vi "test Create Map from Messages to Value Indexes.vi"(8 "error in (no error)":errorcluster, 11 "TestCase in":refnum<class "Engine.lvclass">) -> (0 "error out":errorcluster, 3 "TestCase out":refnum<class "Engine.lvclass">)   [LabVIEW 2020, in "Engine.lvclass"]
uses:
  Engine.lvclass
  Shared/1553 Channel.ctl
  Shared/Terminal Name and Address.ctl
  Shared/Address.ctl
  Shared/Message Definition.ctl
  Shared/Message Type.ctl
  Shared/Terminal Endpoint.ctl
  Shared/Parameter Definition.ctl
  Shared/Map of Messages to Value Indexes.ctl
  Shared/Message Map Key.ctl
  <vilib>/addons/_JKI Toolkits/VI Tester/TestCase.llb/TestCase.lvclass
  Engine/Custom Device/Custom Device.lvlib
  C:/Program Files (x86)/National Instruments/LabVIEW 2020/vi.lib/addons/_JKI Toolkits/VI Tester/TestCase.llb/TestCase.lvclass
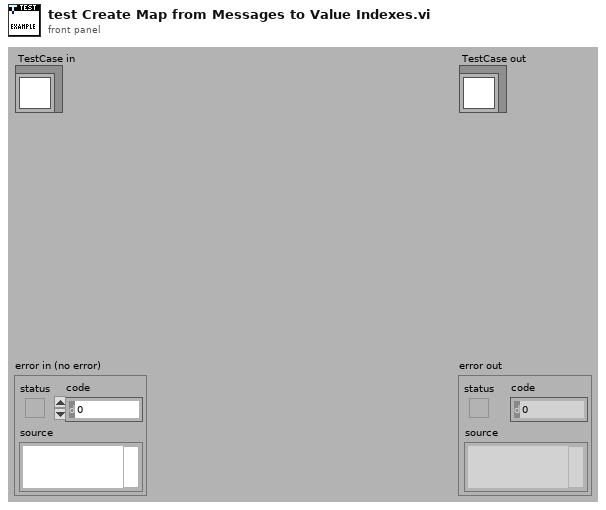
[diagram p1: front panel]
types:
  T1 = typedef "Map of Messages to Value Indexes.ctl" = map{T2, i32}
  T2 = typedef "Message Map Key.ctl" = cluster{"HW channel":u16, "terminal address":u16, "subaddress":u16, "mode code":u16}
  T3 = typedef "1553 Channel.ctl" = cluster{"HW channel":u16, "terminals":T4[], "messages":T6[], "acyclic frame names":string[]}
  T4 = typedef "Terminal Name and Address.ctl" = cluster{"name":string, "terminal address":T5}
  T5 = typedef "Address.ctl" = u16
  T6 = typedef "Message Definition.ctl" = cluster{"name":string, "message type":T7, "endpoint Rx":T8, "endpoint Tx":T8, "mode code":u16, "number of words":u16, "parameters":cluster{"name":string, "default value":dbl, "unit":string, "parameter definition":T9}[], "create timestamp channel":bool}
  T7 = typedef "Message Type.ctl" = string
  T8 = typedef "Terminal Endpoint.ctl" = cluster{"terminal address":T5, "subaddress":T5}
  T9 = typedef "Parameter Definition.ctl" = cluster{"start index":i32, "size (bits)":i32, "encoding":enum16{"BNR", "BCD", "Discrete"}, "signed":bool, "multiplier":dbl, "offset":dbl}
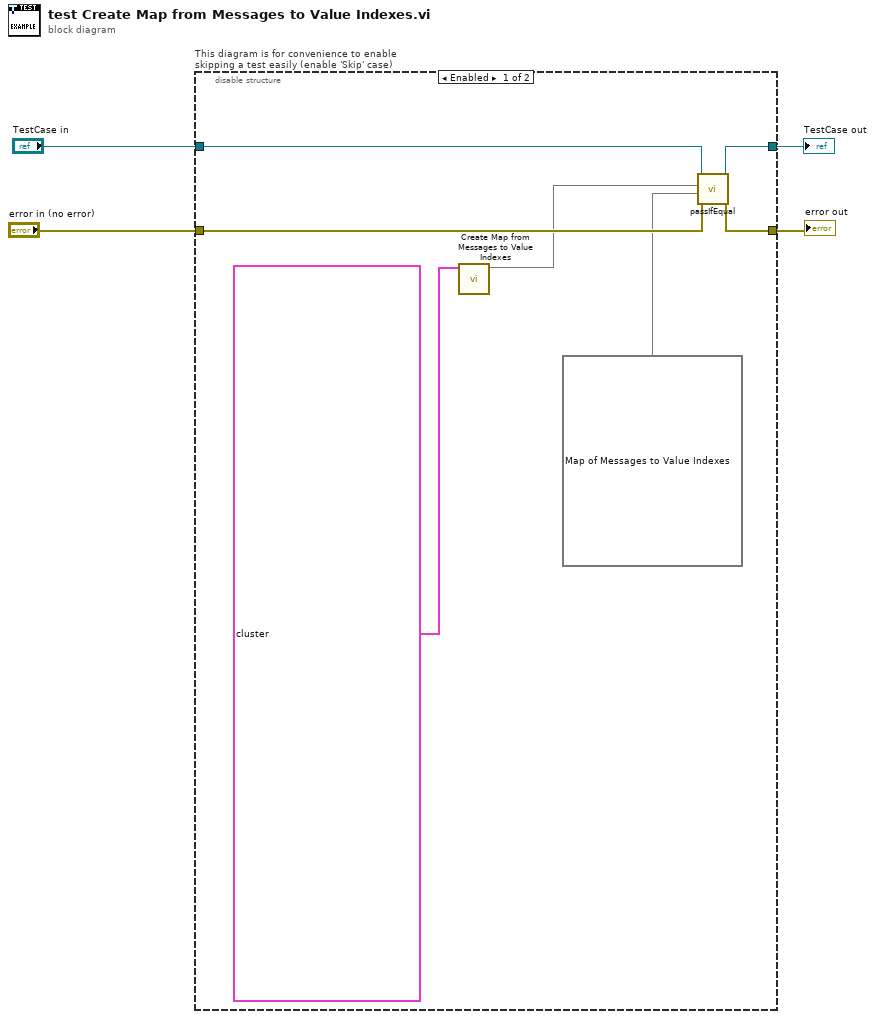
[diagram p0: block diagram]
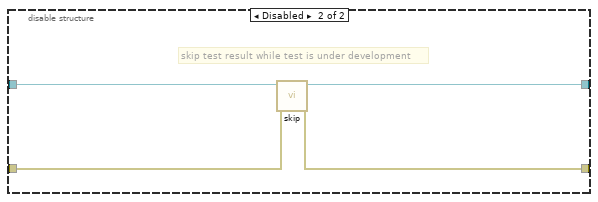
[diagram p2: hidden frame]
diagram:
  n1 = disable-structure "This diagram is for convenience to enable skipping a test easily (enable 'Skip' case)" shown="Enabled" {
    disable-tunnel: "TestCase in" -> [w11 w15]
    disable-tunnel: [w10 w13] -> w1
    disable-tunnel: [w9 w14] -> w3
    disable-tunnel: "error in (no error)" -> [w8 w12]
    frame Enabled {
      n2 = call "Create Map from Messages to Value Indexes.vi"("1553 channels"=T3[] [{"HW channel"=0, "terminals"=[], "messages"=[{"name"="", "message type"="BC to RT", "endpoint Rx"={"terminal address"=1, "subaddress"=2}, "endpoint Tx"={"terminal address"=0, "subaddress"=0}, "mode code"=0, "number of words"=3, "parameters"=[], "create timestamp channel"=FALSE}, {"name"="", "message type"="RT to RT", "endpoint Rx"={"terminal address"=31, "subaddress"=21}, "endpoint Tx"={"terminal address"=15, "subaddress"=21}, "mode code"=0, "number of words"=11, "parameters"=[], "create timestamp channel"=FALSE}, {"name"="", "message type"="BC to RT", "endpoint Rx"={"terminal address"=1, "subaddress"=3}, "endpoint Tx"={"terminal address"=0, "subaddress"=0}, "mode code"=0, "number of words"=4, "parameters"=[], "create timestamp channel"=FALSE}, {"name"="", "message type"="RT to BC", "endpoint Rx"={"terminal address"=0, "subaddress"=0}, "endpoint Tx"={"terminal address"=1, "subaddress"=5}, "mode code"=0, "number of words"=6, "parameters"=[], "create timestamp channel"=FALSE}, {"name"="", "message type"="RT to BC", "endpoint Rx"={"terminal address"=0, "subaddress"=0}, "endpoint Tx"={"terminal address"=1, "subaddress"=6}, "mode code"=0, "number of words"=2, "parameters"=[], "create timestamp channel"=FALSE}, {"name"="", "message type"="RT to RT", "endpoint Rx"={"terminal address"=15, "subaddress"=20}, "endpoint Tx"={"terminal address"=1, "subaddress"=20}, "mode code"=0, "number of words"=4, "parameters"=[], "create timestamp channel"=FALSE}, {"name"="", "message type"="MC", "endpoint Rx"={"terminal address"=0, "subaddress"=0}, "endpoint Tx"={"terminal address"=1, "subaddress"=31}, "mode code"=16, "number of words"=0, "parameters"=[], "create timestamp channel"=FALSE}, {"name"="", "message type"="MC", "endpoint Rx"={"terminal address"=1, "subaddress"=31}, "endpoint Tx"={"terminal address"=0, "subaddress"=0}, "mode code"=17, "number of words"=0, "parameters"=[], "create timestamp channel"=FALSE}, {"name"="", "message type"="BC to RT", "endpoint Rx"={"terminal address"=31, "subaddress"=28}, "endpoint Tx"={"terminal address"=0, "subaddress"=0}, "mode code"=0, "number of words"=6, "parameters"=[], "create timestamp channel"=FALSE}, {"name"="", "message type"="MC", "endpoint Rx"={"terminal address"=31, "subaddress"=31}, "endpoint Tx"={"terminal address"=0, "subaddress"=0}, "mode code"=1, "number of words"=0, "parameters"=[], "create timestamp channel"=FALSE}], "acyclic frame names"=[]}]) -> ("map from messages to value indexes"=w7:T1)  [unwired: 10 in]
      n3 = call-dynamic "passIfEqual.vi"("error in (no error)"=w8, "y"=T1 {{"HW channel"=0, "terminal address"=1, "subaddress"=2, "mode code"=0}=0, {"HW channel"=0, "terminal address"=1, "subaddress"=3, "mode code"=0}=14, {"HW channel"=0, "terminal address"=1, "subaddress"=5, "mode code"=0}=18, {"HW channel"=0, "terminal address"=1, "subaddress"=6, "mode code"=0}=24, {"HW channel"=0, "terminal address"=1, "subaddress"=31, "mode code"=16}=30, {"HW channel"=0, "terminal address"=1, "subaddress"=31, "mode code"=17}=31, {"HW channel"=0, "terminal address"=15, "subaddress"=20, "mode code"=0}=26, {"HW channel"=0, "terminal address"=31, "subaddress"=21, "mode code"=0}=3, {"HW channel"=0, "terminal address"=31, "subaddress"=28, "mode code"=0}=32, {"HW channel"=0, "terminal address"=31, "subaddress"=31, "mode code"=1}=38} ("map from messages to value indexes"), "x"=w7, "TestCase in"=w11) -> ("error out"=w9:errorcluster, "TestCase out"=w10:refnum<class "Engine.lvclass">)  [unwired: 6 in]
    }
    frame Disabled {
      # "skip test result while test is under development"
      n4 = call <vilib>:"skip.vi"("error in (no error)"=w12, "TestCase in"=w15) -> ("error out"=w14:errorcluster, "TestCase out"=w13:refnum<class "Engine.lvclass">)  [unwired: 8 in]
    }
  }
  "error out" <- w3
  "TestCase out" <- w1
